vi "DAQ - WRITE - Simple digital pulse.vi"(8 "error in":errorcluster, 10 "data":bool, 11 "task/channels in":refnum<k21>) -> (0 "error out":errorcluster, 3 "task out":refnum<k21>)   [LabVIEW 2017]
uses:
  <vilib>/DAQmx/write.llb/DAQmx Write (Digital Bool 1Line 1Point).vi
  <vilib>/DAQmx/miscellaneous.llb/DAQmx Fill In Error Info.vi
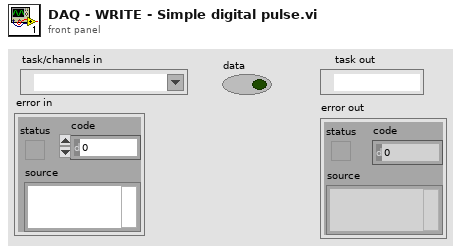
[diagram p1: front panel]
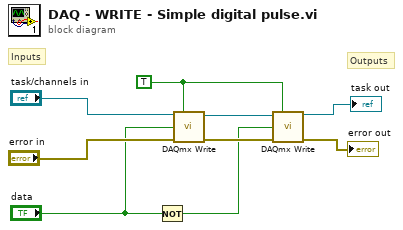
[diagram p0: block diagram]
diagram:
  w3 = TRUE ("auto start")
  # "Outputs"
  # "Inputs"
  n1 = Not(x="data") -> (.not. x?=w2:bool)
  n2 = call-poly <vilib>:"DAQmx Write.vi"("task/channels in"="task/channels in", "auto start"=w3, "data"="data", "error in"="error in") -> ("task out"=w9:refnum<k21>, "error out"=w4:errorcluster)  [unwired: 9 in, 1 out]
  n3 = call-poly <vilib>:"DAQmx Write.vi"("task/channels in"=w9, "auto start"=w3, "data"=w2, "error in"=w4) -> ("task out"=→"task out":refnum<k21>, "error out"=→"error out":errorcluster)  [unwired: 9 in, 1 out]
